vi "Set Frame Array File Needed Property.vi"(8 "error in":errorcluster, 10 "needed?":bool, 11 "custom device ref in":T1 format="%.0x") -> (0 "error out":errorcluster, 3 "custom device ref out":T1 format="%.0x")   [LabVIEW 2020, in "AIM ARINC 664 Scripting.lvlib"]
uses:
  AIM ARINC 664 Scripting.lvlib
  Constants.vi
  <vilib>/NI VeriStand/Custom Device API/Custom Device API.lvlib
  <vilib>/NI VeriStand/Custom Device Tools/Custom Device Utility Library/Custom Device Utility Library.lvlib
  <vilib>/NI VeriStand/Custom Device Tools/Custom Device Utility Library/NI VeriStand - Search for Item by GUID.vi
  <vilib>/NI VeriStand/Custom Device API/Set Item Property (Boolean).vi
  <vilib>/NI VeriStand/Custom Device API/Custom Device Item Ref.ctl
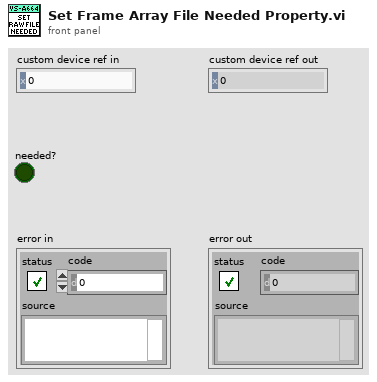
[diagram p1: front panel]
types:
  T1 = typedef "Custom Device API.lvlib/Custom Device Item Ref.ctl" = u64
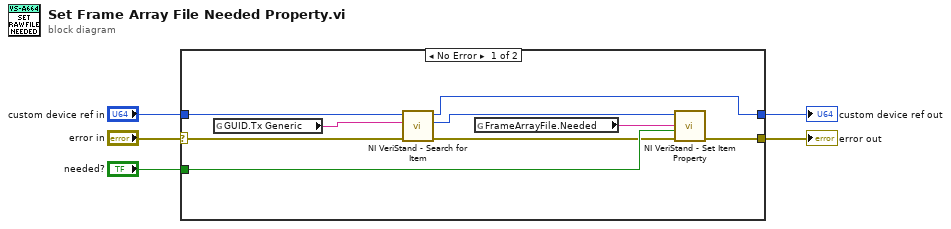
[diagram p0: block diagram]
diagram:
  n1 = case shown="No Error" "error in" {
    selector: "error in" -> [w14 w16]
    tunnel: "custom device ref in" -> [w8 w15]
    tunnel: [w13 w16] -> w4
    tunnel: [w7 w15] -> w3
    tunnel: "needed?" -> [w11 _]
    frame No Error {
      n2 = global read "Constants.vi" "GUID.Tx Generic"() -> (w6:string)
      n3 = call-poly <vilib>:"NI VeriStand - Search for Item.vi"("error in"=w14, "Item GUID"=w6, "Section Ref in"=w8) -> ("error out"=w10:errorcluster, "Item Ref"=w9:T1, "Section Ref out"=w7:T1)  [unwired: 5 in, 1 out]
      n4 = global read "Constants.vi" "FrameArrayFile.Needed"() -> (w12:string)
      n5 = call-poly <vilib>:"NI VeriStand - Set Item Property.vi"("error in (no error)"=w10, "Value"=w11, "Property Name"=w12, "Item Ref in"=w9) -> ("error out"=w13:errorcluster)  [unwired: 5 in, 2 out]
    }
    frame Error {
    }
  }
  "error out" <- w4
  "custom device ref out" <- w3
